vi "conversion_rad_to_rpm.vi"(1 "x (rad/s)":dbl) -> (0 "x (rpm)":dbl)   [LabVIEW 2021]
doc: "Converts rad/s to rpm."
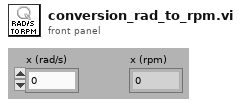
[diagram p1: front panel]
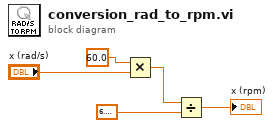
[diagram p0: block diagram]
diagram:
  n1 = Multiply(x=60.0 ("y"), y="x (rad/s)") -> (x*y=w1:dbl)
  n2 = Divide(x=w1, y=6.283185307179586) -> (x/y=→"x (rpm)":dbl)
